vi "VI Tree - JKI State Machine__jki_lib_state_machine.vi"   [LabVIEW 2010]
panel:
  # "VI TREE"
  # "For instructions on how to use the JKI State Machine, examples and video tutorials, visit:\nhttp://jkisoft.com/state-machine/\n\nJKI State Machine™\nhttp://jkisoft.com/state-machine/\nCopyright (C) 2005-2008, JKI <info@jkisoft.com>\nALL RIGHTS RESERVED"
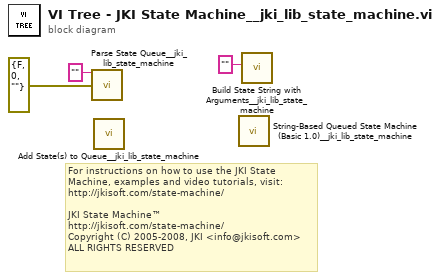
[diagram p0: block diagram]
diagram:
  # "For instructions on how to use the JKI State Machine, examples and video tutorials, visit:\nhttp://jkisoft.com/state-machine/\n\nJKI State Machine™\nhttp://jkisoft.com/state-machine/\nCopyright (C) 2005-2008, JKI <info@jkisoft.com>\nALL RIGHTS RESERVED"
  n1 = call "Parse State Queue__jki_lib_state_machine.vi"("State Queue"="", "Error In (no error)"=errorcluster {"status"=FALSE, "code"=0, "source"=""} ("Error")) -> ()  [unwired: 11 in, 3 out]
  n2 = call "Add State(s) to Queue__jki_lib_state_machine.vi"() -> ()  [unwired: 15 in, 1 out]
  n3 = call "String-Based Queued State Machine (Basic 1.0)__jki_lib_state_machine.vi"() -> ()  [unwired: 1 in]
  n4 = call "Build State String with Arguments__jki_lib_state_machine.vi"("State"="" ("State (\"\")")) -> ()  [unwired: 5 in, 1 out]
